vi "Robot Global Reference.vi"() -> ()   [LabVIEW 2016]
uses:
  Global References.ctl
  Joystick Reference.ctl
  <vilib>/Rock Robotics/WPI/Joystick/WPI_JoystickDevRef.ctl
  <vilib>/Rock Robotics/WPI/Joystick/WPI_JoystickDeviceEnum.ctl
  Drive Reference.ctl
  <vilib>/Rock Robotics/WPI/RobotDrive/WPI_RobotDriveDevRef.ctl
  <vilib>/Rock Robotics/WPI/MotorControl/WPI_MotorControlDeviceRef.ctl
  <vilib>/Rock Robotics/WPI/MotorControl/WPI_MotorControlType.ctl
  <vilib>/Rock Robotics/SystemInterfaces/DIO/FPGA_DIOPWMChannel.ctl
  <vilib>/Rock Robotics/WPI/PWM/WPI_PWMDeadband.ctl
  Sensor Reference.ctl
  Acquisition Reference.ctl
  Shoot Reference.ctl
panel:
  in  "Global References":T1={"Joystick Reference"={"Driver Joystick"={"Device"=enum."USB 0"}, "Operator Joystick"={"Device"=enum."USB 0"}}, "Drive Reference"={"RobotDriveDevRef"={"DevStatus"={"status"=FALSE, "code"=0, "source"=""}, "Motors[]"=[], "Square Inputs"=FALSE, "Max Output"=1.0}}, "Sensor Reference"={"This is a\nplaceholder,\nadd references\nas needed."=FALSE}, "Acquisition Reference"={"This is a\nplaceholder,\nadd references\nas needed."=FALSE}, "Shoot Reference"={"This is a\nplaceholder,\nadd references\nas needed."=FALSE}}
  # "Placeholders are needed or else\nthe project will not compile."
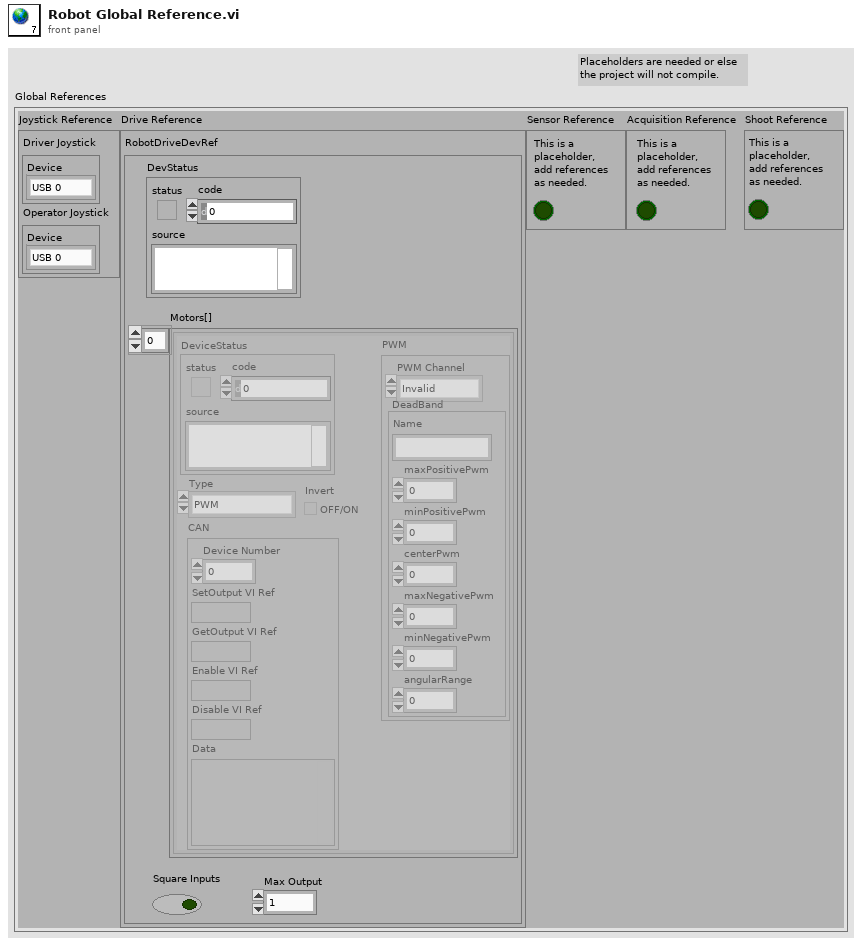
[diagram p1: front panel]
types:
  T1 = typedef "Global References.ctl" = cluster{"Joystick Reference":T2, "Drive Reference":T5, "Sensor Reference":T11, "Acquisition Reference":T12, "Shoot Reference":T13}
  T2 = typedef "Joystick Reference.ctl" = cluster{"Driver Joystick":T3, "Operator Joystick":T3}
  T3 = typedef "WPI_JoystickDevRef.ctl" = cluster{"Device":T4}
  T4 = typedef "WPI_JoystickDeviceEnum.ctl" = enum16{"USB 0", "USB 1", "USB 2", "USB 3", "USB 4", "USB 5"}
  T5 = typedef "Drive Reference.ctl" = cluster{"RobotDriveDevRef":T6}
  T6 = typedef "WPI_RobotDriveDevRef.ctl" = cluster{"DevStatus":errorcluster, "Motors[]":T7[], "Square Inputs":bool, "Max Output":dbl}
  T7 = typedef "WPI_MotorControlDeviceRef.ctl" = cluster{"DeviceStatus":errorcluster, "Type":T8, "PWM":cluster{"PWM Channel":T9, "DeadBand":T10}, "CAN":cluster{"Device Number":u8, "SetOutput VI Ref":variant, "GetOutput VI Ref":variant, "Enable VI Ref":variant, "Disable VI Ref":variant, "Data":variant}, "Invert":bool}
  T8 = typedef "WPI_MotorControlType.ctl" = enum16{"PWM", "CAN"}
  T9 = typedef "FPGA_DIOPWMChannel.ctl" = enum8{"PWM 0", "PWM 1", "PWM 2", "PWM 3", "PWM 4", "PWM 5", "PWM 6", "PWM 7", "PWM 8", "PWM 9", "PWM MXP 0", "PWM MXP 1", "PWM MXP 2", "PWM MXP 3", "PWM MXP 4", "PWM MXP 5", "PWM MXP 6", "PWM MXP 7", "PWM MXP 8", "PWM MXP 9", "Invalid"}
  T10 = typedef "WPI_PWMDeadband.ctl" = cluster{"Name":string, "maxPositivePwm":i32, "minPositivePwm":i32, "centerPwm":i32, "maxNegativePwm":i32, "minNegativePwm":i32, "angularRange":u16}
  T11 = typedef "Sensor Reference.ctl" = cluster{"This is a\nplaceholder,\nadd references\nas needed.":bool}
  T12 = typedef "Acquisition Reference.ctl" = cluster{"This is a\nplaceholder,\nadd references\nas needed.":bool}
  T13 = typedef "Shoot Reference.ctl" = cluster{"This is a\nplaceholder,\nadd references\nas needed.":bool}
diagram:
